vi "UIRef.vi"(8 "error in":errorcluster, 11 "node in":refnum<class "Pages.lvclass">) -> (0 "error out":errorcluster, 2 "VI refnum":refnum<vi>, 3 "node out":refnum<class "Pages.lvclass">)   [LabVIEW 2019, in "Pages.lvclass"]
doc: "Stores the static reference to the UI of the node."
uses:
  Pages.lvclass
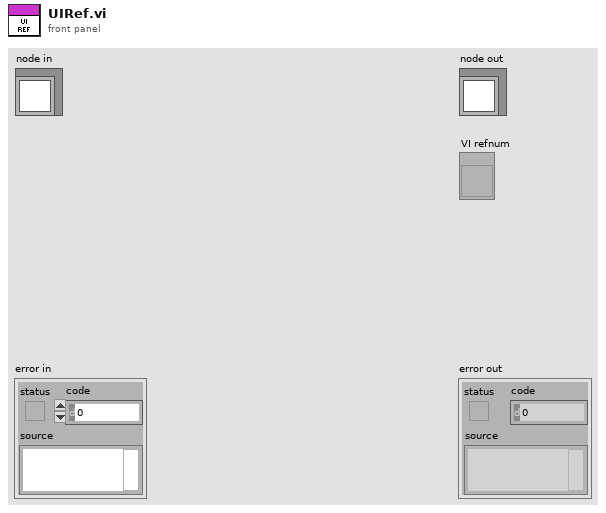
[diagram p1: front panel]
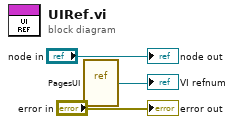
[diagram p0: block diagram]
diagram:
  n1 = vi-ref "PagesUI.vi"() -> (→"VI refnum":refnum<vi>)
  "error out" <- "error in"
  "node out" <- "node in"
